vi "Read Floor Selection.vi"(8 "error in (no error)":errorcluster, 11 "Sim User Console Actor in":refnum<class "Sim User Console Actor.lvclass">) -> (0 "error out":errorcluster, 2 "Floor Selection":refnum<vi>, 3 "Sim User Console Actor out":refnum<class "Sim User Console Actor.lvclass">)   [LabVIEW 2022 SP3, in "Sim User Console Actor.lvlib" / "Sim User Console Actor.lvclass"]
uses:
  Sim User Console Actor.lvclass
  Sim User Console Actor.lvclass/Sim User Console Actor.ctl
  Abstract User Console Actor/Abstract User Console Actor/Floor Selection.ctl
  Abstract User Console Actor/Abstract User Console Actor/Abstract User Console Actor.lvclass
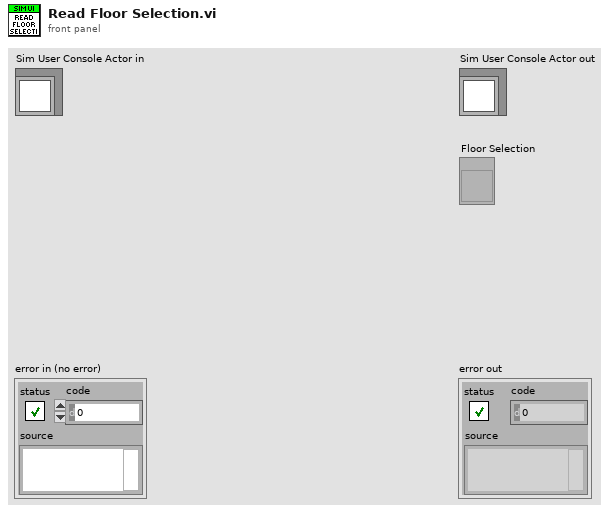
[diagram p1: front panel]
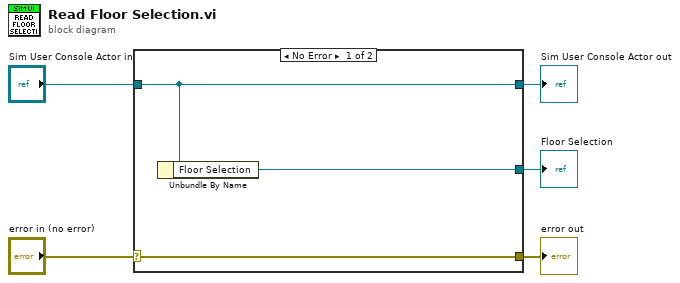
[diagram p0: block diagram]
diagram:
  n1 = case shown="No Error" "error in (no error)" {
    selector: "error in (no error)" -> [w8 w9]
    tunnel: [w8 w9] -> w4
    tunnel: [w7 w10] -> w2
    tunnel: "Sim User Console Actor in" -> [w7 w10]
    tunnel: [w6 _] -> w1
    frame No Error {
      n2 = Unbundle By Name(w7) -> ("Floor Selection"=w6:refnum<vi>)
    }
    frame Error {
    }
  }
  "error out" <- w4
  "Sim User Console Actor out" <- w2
  "Floor Selection" <- w1
